vi "2022_day3.vi"() -> ()   [LabVIEW 2021]
uses:
  <vilib>/WebDAVClient/Simple Get Buffer.vi
  <vilib>/WebDAVClient/NI_WebDAV.lvlib
panel:
  out "Task 2":i32
  out "Task 1":i32
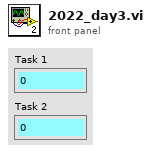
[diagram p1: front panel]
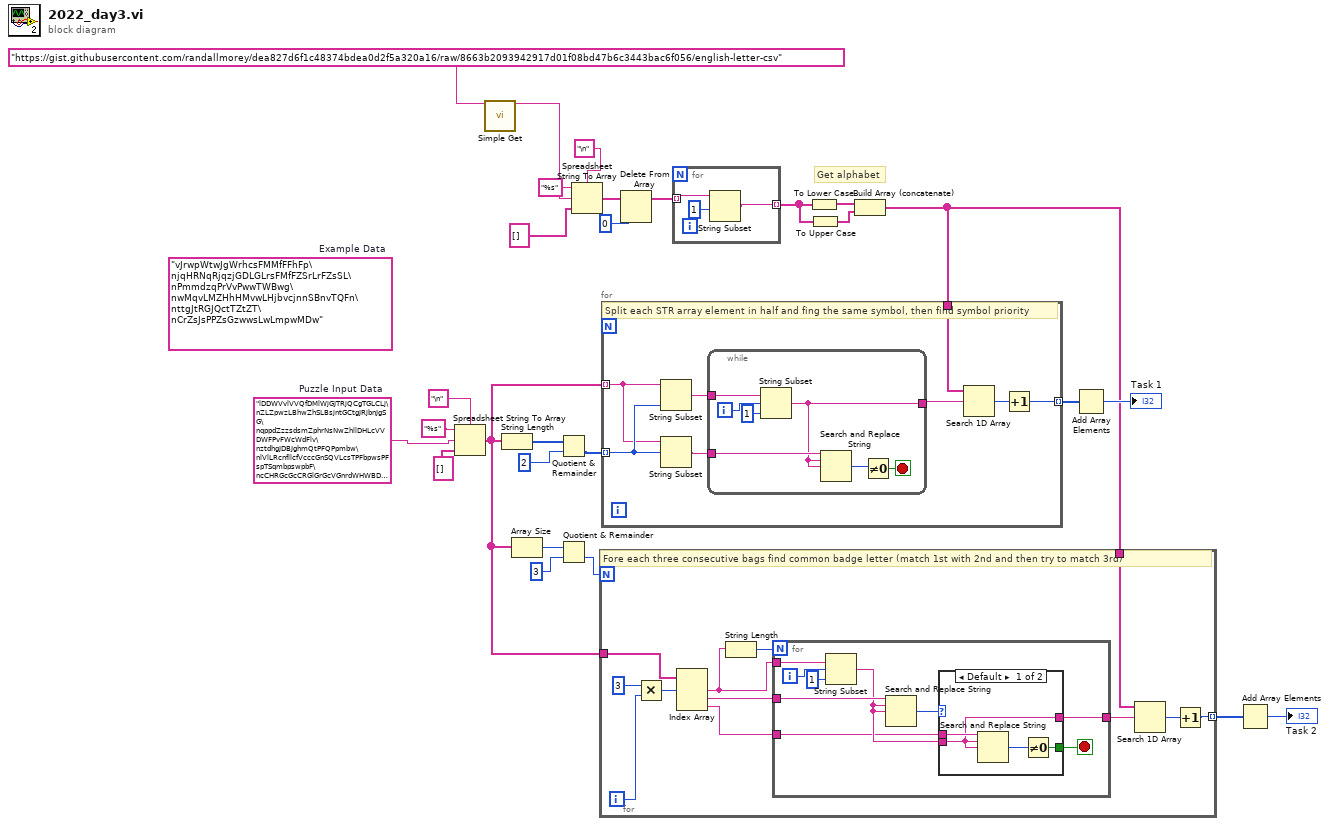
[diagram p0: block diagram]
diagram:
  w1 = "lDDWVvlVVQfDMlWjGJTRjQCgTGLCLj\nZLZpwzLBhwZhSLBsjntGCtgJRjbnJgSG\nqppdZzzsdsmZphrNsNwZhllDHLcVVDWFPvFWcWdFlv\nztdhgJDBJghmQtPFQPpmbw\nlVlLRcnfllcfVcccGnSQVLcsTPFbpwsPFspTSqmbpswpbF\ncCHRGcGcCRGlGrGcVGnrdWHWBDzBNhhQZWWNBhJz\nNfnSSQpdnRSSpvWdSsjZDGNDjGDwTGTjHG\nwlPzPqzPFbMmqPCFCJmbsjbHLDDHDZjDjbGHsT\ngwMlgmtmPcqVVvhVnvcRnn\ncBNBBCHhbhNhblBcCCvcBHSwTwDQSqRwDQpDRsjHST\ndPmzMVWdmmMnnZJtZVdqjTSrjTjrpQrsTTVwQRSj\nqzmZMmdZPtnGqclblGlbGvgBFc\nZfpmNDfRhzbbqDnD\nSFtFjTTZVTFvVTjHrsVvqGBJqhnSSnbJznLGJwJq\nTjdPPtdMPPWCcZgW\nqsbmGCsjHNhmhmhzTDznpnlQZlbWlZ\nLTSSfSvggVVgBgfLtvvtTSczzpWnZQZnlnzpBcnWpQWc\nFrLvrrrVPgdPftSHHdNsjTH..."  # Puzzle Input Data
  (unwired) "vJrwpWtwJgWrhcsFMMfFFhFp\njqHRNqRjqzjGDLGLrsFMfFZSrLrFZsSL\nPmmdzqPrVvPwwTWBwg\nwMqvLMZHhHMvwLHjbvcjnnSBnvTQFn\nttgJtRGJQctTZtZT\nCrZsJsPPZsGzwwsLwLmpwMDw"  # Example Data
  # "Get alphabet"
  n1 = Spreadsheet String To Array(delimiter (Tab)="\n", format string="%s", spreadsheet string=w1, array type (2D Dbl)=string[] []) -> (array=w3:string[])
  n2 = call-poly <vilib>:"Simple Get.vi"("remote file uri"="https://gist.githubusercontent.com/randallmorey/dea827d6f1c48374bdea0d2f5a320a16/raw/8663b2093942917d01f08bd47b6c3443bac6f056/english-letter-csv") -> ("data"=w26:string)  [unwired: 13 in, 1 out]
  n3 = String Length(string=w3) -> (length=w5:i32[])
  n4 = Array Size(array=w3) -> (size(s)=w2:i32)
  n5 = Quotient & Remainder(x=w5, y=2 ("format string")) -> (floor(x/y)=w12:i32[])  [unwired: 1 out]
  n6 = Quotient & Remainder(x=w2, y=3 ("format string")) -> (floor(x/y)=w4:i32)  [unwired: 1 out]
  n7 = Spreadsheet String To Array(delimiter (Tab)="\n", format string="%s", spreadsheet string=w26, array type (2D Dbl)=string[] []) -> (array=w22:string[])
  n8 = Delete From Array(array=w22, index=0) -> (array with subset deleted=w21:string[])  [unwired: 1 in, 1 out]
  n9 = for {
    tunnel: w21 -> [w30] mode=indexing
    tunnel: [w28] -> w19 mode=indexing
    n10 = String Subset(string=w30, length (rest)=1 ("length (rest)")) -> (substring=w28:string)  [unwired: 1 in]
  }
  n11 = To Lower Case(string=w19) -> (all lower case string=w18:string[])
  n12 = To Upper Case(1:w19) -> (0:w17:string[])
  n13 = Build Array (concatenate)(w18, w17) -> (w9:string[])
  n14 = for {
    N: w4 -> [_]
    tunnel: w3 -> [w40]
    tunnel: w9 -> [w32]
    tunnel: [w31] -> w7 mode=indexing
    i -> [w42]
    # "Fore each three consecutive bags find common badge letter (match 1st with 2nd and then try to match 3rd)"
    n15 = Multiply(x=3, y=w42) -> (x*y=w39:i32)
    n16 = Index Array(array=w40, index #1=w39) -> (element #1=w36:string, element #2=w38:string, element #3=w35:string)  [unwired: 2 in]
    n17 = String Length(string=w36) -> (length=w37:i32)
    n18 = for {
      N: w37 -> [_]
      tunnel: w36 -> [w51]
      tunnel: w38 -> [w48]
      tunnel: w35 -> [w45]
      tunnel: [w43] -> w33
      i -> [w50]
      stop <- w44 stop-if-true
      n19 = String Subset(string=w51, offset (0)=w50, length (rest)=1 ("length (rest)")) -> (substring=w46:string)
      n20 = Search and Replace String(input string=w48, search string=w46, replace string=w46) -> (number of replacements=w47:i32)  [unwired: 5 in, 3 out]
      n21 = case shown="Default" w47 {
        tunnel: w46 -> [w52 _]
        tunnel: w45 -> [w55 _]
        tunnel: [w53 _] -> w44
        tunnel: [w52 _] -> w43
        frame Default {
          n22 = Search and Replace String(input string=w55, search string=w52, replace string=w52) -> (number of replacements=w54:i32)  [unwired: 5 in, 3 out]
          n23 = Not Equal To 0?(x=w54) -> (x != 0?=w53:bool)
        }
        frame 0 {
        }
      }
    }
    n24 = Search 1D Array(1D array=w32, element=w33) -> (index of element=w34:i32)  [unwired: 1 in]
    n25 = Increment(x=w34) -> (x+1=w31:i32)
  }
  n26 = for {
    tunnel: w12 -> [w63] mode=indexing
    tunnel: w3 -> [w62] mode=indexing
    tunnel: w9 -> [w59]
    tunnel: [w56] -> w11 mode=indexing
    # "Split each STR array element in half and fing the same symbol, then find symbol priority"
    n27 = String Subset(string=w62, length (rest)=w63) -> (substring=w60:string)  [unwired: 1 in]
    n28 = String Subset(string=w62, offset (0)=w63) -> (substring=w61:string)  [unwired: 1 in]
    n29 = while {
      tunnel: w61 -> [w67]
      tunnel: w60 -> [w70]
      tunnel: [w64] -> w58
      i -> [w69]
      stop <- w65 stop-if-true
      n30 = String Subset(string=w70, offset (0)=w69, length (rest)=1 ("length (rest)")) -> (substring=w64:string)
      n31 = Search and Replace String(input string=w67, search string=w64, replace string=w64) -> (number of replacements=w66:i32)  [unwired: 5 in, 3 out]
      n32 = Not Equal To 0?(x=w66) -> (x != 0?=w65:bool)
    }
    n33 = Search 1D Array(1D array=w59, element=w58) -> (index of element=w57:i32)  [unwired: 1 in]
    n34 = Increment(x=w57) -> (x+1=w56:i32)
  }
  n35 = Add Array Elements(numeric array=w11) -> (sum=→"Task 1":i32)
  n36 = Add Array Elements(numeric array=w7) -> (sum=→"Task 2":i32)
